vi "Coordinates to Multicolumn Listbox Column.vi"(9 "Coords":T1, 11 "MulticolumnListbox in":refnum<vi>) -> (3 "Column":i32)   [LabVIEW 2020, in "TdmsFileViewer.lvlib"]
uses:
  TdmsFileViewer.lvlib
  <vilib>/Utility/miscctls.llb/LVPoint32TypeDef.ctl
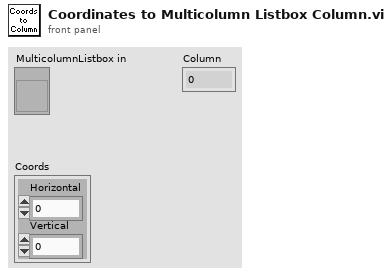
[diagram p1: front panel]
types:
  T1 = typedef "LVPoint32TypeDef.ctl" = cluster{"Horizontal":i32, "Vertical":i32}
  T2 = typedef "LVRowAndColumnTypeDef.ctl" = cluster{"Row":i32, "Column":i32}
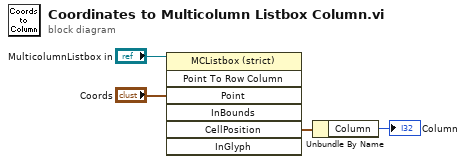
[diagram p0: block diagram]
diagram:
  n1 = invoke on="Invoke Node" class="MCListbox (strict)" method="Point To Row Column"(reference="MulticolumnListbox in", "Point"="Coords") -> ("CellPosition"=w3:T2)  [unwired: 5 in, 6 out]
  n2 = Unbundle By Name(w3) -> ("Column"=→"Column":i32)
